vi "test_udp_read.vi"() -> ()   [LabVIEW 2019]
uses:
  <vilib>/Utility/tcp.llb/UDP Multicast Read-Only Open.vi
panel:
  out "TopIpAddr":string
  out "TopTCPPort":u16
  out "error out":errorcluster
  out "data out":string
  in  "TopUDPPort":u16
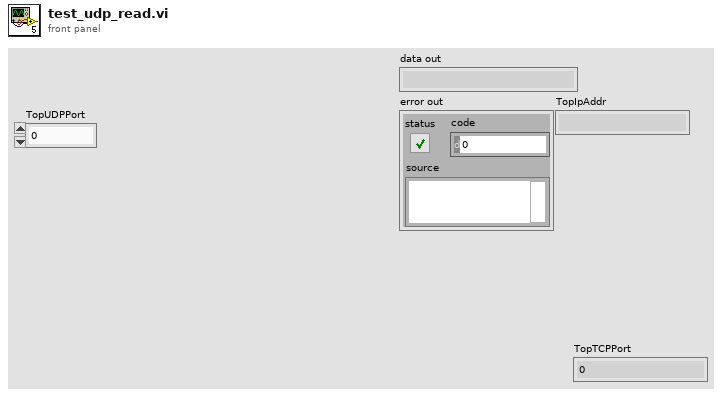
[diagram p1: front panel]
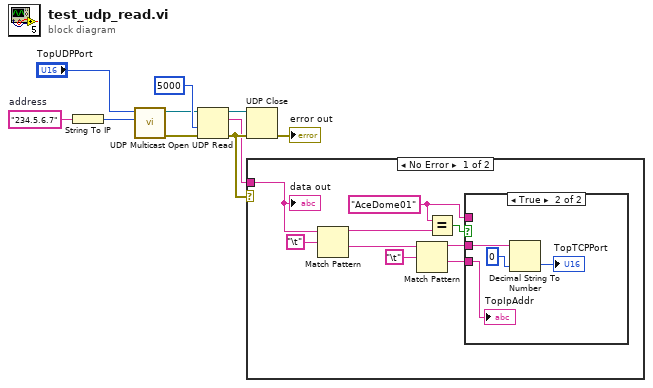
[diagram p0: block diagram]
diagram:
  w10 = "234.5.6.7"  # address
  n1 = String To IP(1:w10) -> (0:w9:u32)
  n2 = call-poly <vilib>:"UDP Multicast Open.vi"("multicast addr"=w9, "port"="TopUDPPort") -> ("error out"=w5:errorcluster, "connection ID"=w6:refnum<k16>)  [unwired: 7 in, 1 out]
  n3 = UDP Read(connection ID=w6, timeout ms (25000)=5000, 8:w5) -> (data out=w1:string, error out=w2:errorcluster, 3:w4:refnum<k16>)  [unwired: 1 in, 2 out]
  n4 = UDP Close(connection ID=w4, 8:w2) -> (error out=→"error out":errorcluster)  [unwired: 1 out]
  n5 = case shown="No Error" w2 {
    tunnel: w1 -> [w15 _]
    frame No Error {
      w13 = "AceDome01" ("x")
      n6 = Match Pattern(string=w15, regular expression="\t") -> (before substring=w18:string, after substring=w16:string)  [unwired: 1 in, 2 out]
      n7 = Match Pattern(string=w16, regular expression="\t") -> (before substring=w12:string, after substring=w11:string)  [unwired: 1 in, 2 out]
      n8 = Equal?(x=w13, y=w18) -> (x = y?=w14:bool)
      n9 = case shown="True" w14 {
        tunnel: w13 -> [_ _]
        tunnel: w12 -> [_ w21]
        tunnel: w11 -> [_ w20]
        frame False {
        }
        frame True {
          n10 = Decimal String To Number(string=w21, default (0L)=u16 0) -> (number=→"TopTCPPort":u16)  [unwired: 1 in, 1 out]
          "TopIpAddr" <- w20
        }
      }
      "data out" <- w15
    }
    frame Error {
    }
  }
